vi "Read address.vi"(8 "error in (no error)":errorcluster, 11 "Connection.TCP":refnum<class "Connection.Collection.lvclass">) -> (0 "error out":errorcluster, 2 "address":string="localhost", 3 "Connection.TCP":refnum<class "Connection.Collection.lvclass">)   [LabVIEW 2013]
uses:
  Connection.Collection.lvclass
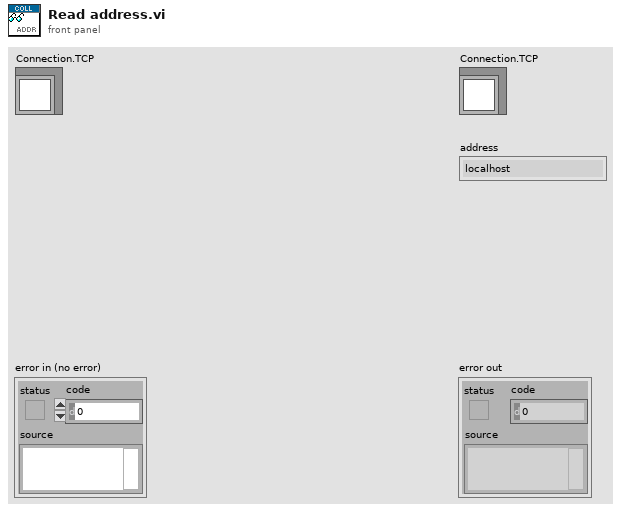
[diagram p1: front panel]
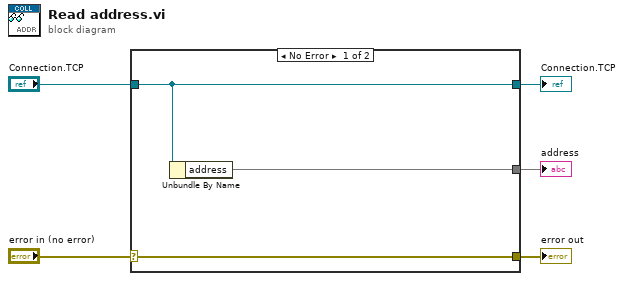
[diagram p0: block diagram]
diagram:
  n1 = case shown="No Error" "error in (no error)" {
    selector: "error in (no error)" -> [w8 w9]
    tunnel: [w8 w9] -> w4
    tunnel: [w7 w10] -> w2
    tunnel: "Connection.TCP" -> [w7 w10]
    tunnel: [w6 _] -> w1
    frame No Error {
      n2 = Unbundle By Name(w7) -> ("address"=w6)
    }
    frame Error {
    }
  }
  "error out" <- w4
  "Connection.TCP" <- w2
  "address" <- w1
